vi "Execute State.vi"(8 "error in (no error)":errorcluster, 10 "System":refnum<class "System.lvclass">, 11 "Command in":refnum<class "Command.lvclass">) -> (0 "error out":errorcluster, 2 "StateExecuteTicks":u32, 3 "Command out":refnum<class "Command.lvclass">)   [LabVIEW 2013, in "Command.lvclass"]
uses:
  Command.lvclass
  Systems/System/System.lvclass
  Command.lvclass/Command.ctl
  States/State/State.lvclass
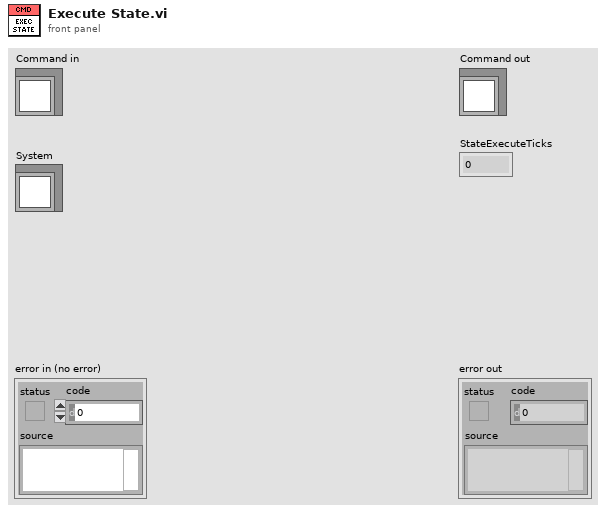
[diagram p1: front panel]
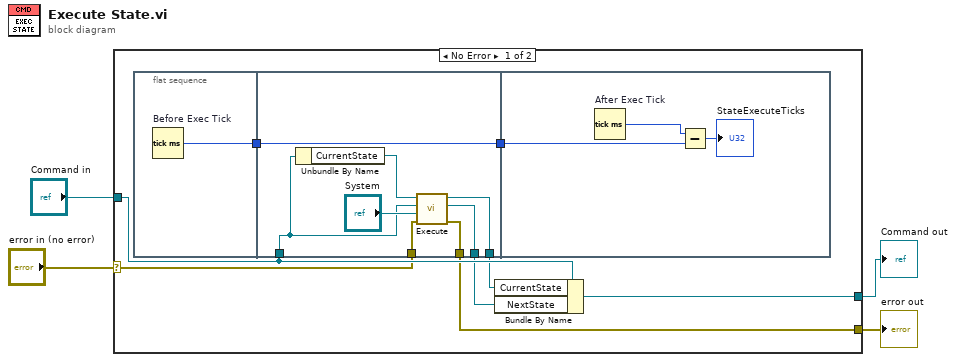
[diagram p0: block diagram]
diagram:
  n1 = case shown="No Error" "error in (no error)" {
    selector: "error in (no error)" -> [w6 w26]
    tunnel: [w5 w26] -> w3
    tunnel: [w9 w25] -> w1
    tunnel: "Command in" -> [w10 w25]
    frame No Error {
      n2 = flat-sequence {
        tunnel: [w13] -> w11
        tunnel: [w20] -> w12
        tunnel: w11 -> [w20]
        tunnel: w10 -> [w18]
        tunnel: [w17] -> w8
        tunnel: [w16] -> w7
        tunnel: w6 -> [w15]
        tunnel: [w14] -> w5
        tunnel: w12 -> [w23]
        frame #0 {
          n3 = Tick Count (ms) "Before Exec Tick"() -> (millisecond timer value=w13:u32)
        }
        frame #1 {
          n4 = Unbundle By Name(w18) -> ("CurrentState"=w19:refnum<class "State.lvclass">)
          n5 = call-dynamic "Execute.vi"("error in (no error)"=w15, "System in"="System", "Command in"=w18, "State in"=w19) -> ("error out"=w14:errorcluster, "Next State"=w16:refnum<class "State.lvclass">, "State out"=w17:refnum<class "State.lvclass">)  [unwired: 5 in]
        }
        frame #2 {
          n6 = Tick Count (ms) "After Exec Tick"() -> (millisecond timer value=w24:u32)
          n7 = Subtract(x=w24, y=w23) -> (x-y=→"StateExecuteTicks":u32)
        }
      }
      n8 = Bundle By Name(cluster=w10, "CurrentState"=w8, "NextState"=w7) -> (w9:refnum<class "Command.lvclass">)
    }
    frame Error {
    }
  }
  "error out" <- w3
  "Command out" <- w1
